vi "Ignore_Channel_evaluate.vi"(7 "Ignore When String":string, 8 "Ignore array":bool[](array[boolean]), 9 "Commands in":string[](array[string]), 10 "Data":string[][](array[string]), 11 "Template Names":string[](array[string])) -> (0 "Ignore array out":bool[](array[boolean]), 1 "Commands Out":string[](array[string]), 3 "Ignore Column":bool)   [LabVIEW 2010]
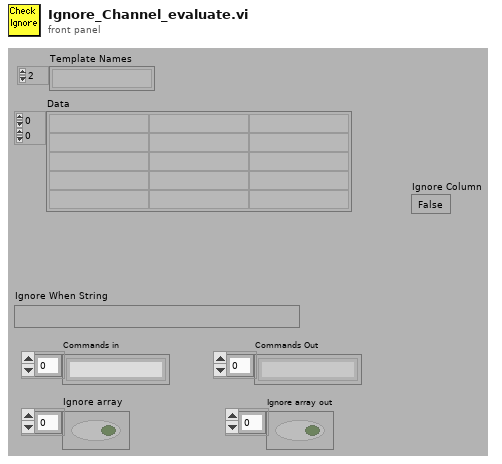
[diagram p1: front panel]
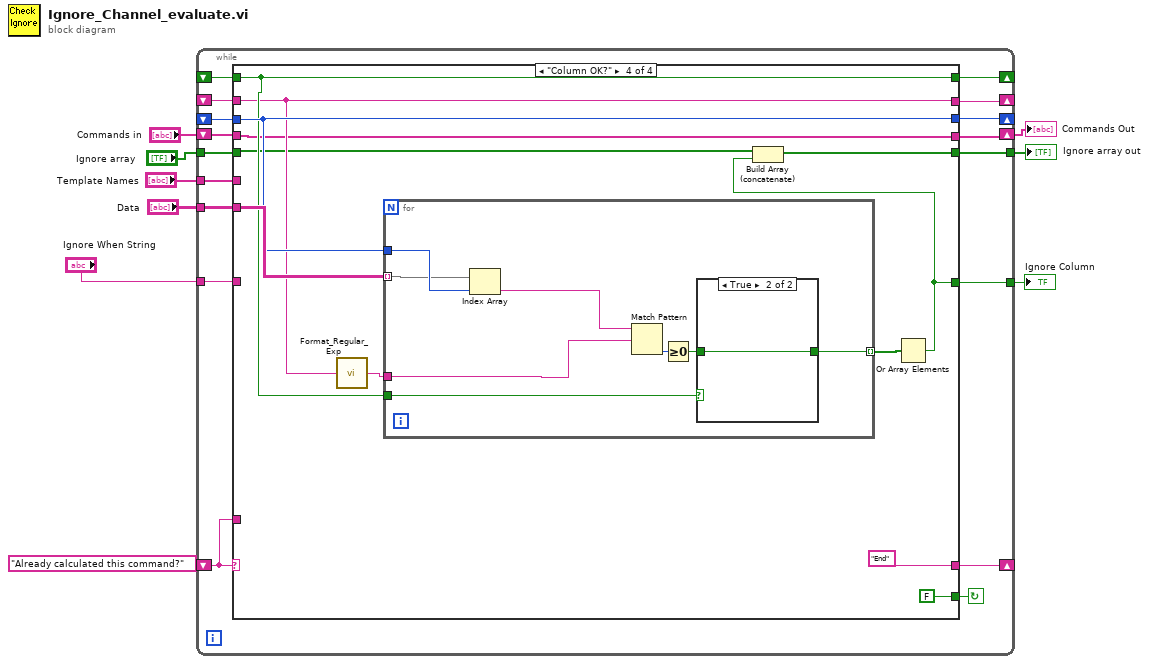
[diagram p0: block diagram]
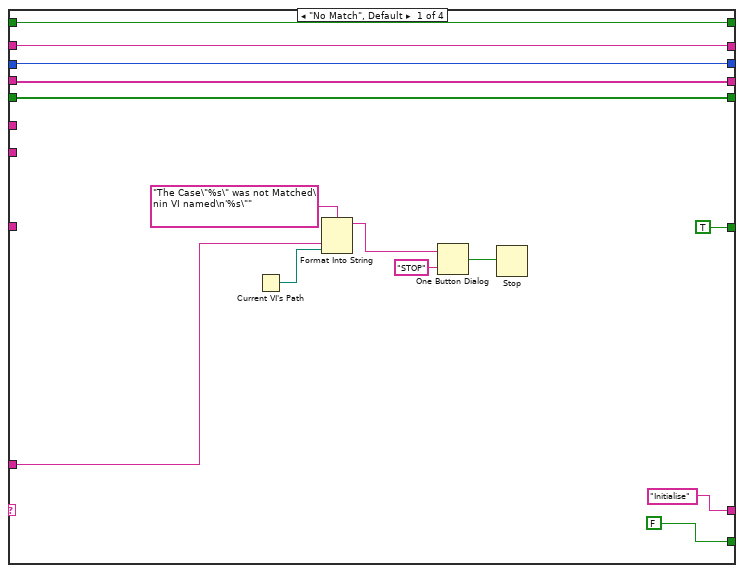
[diagram p2: hidden frame]
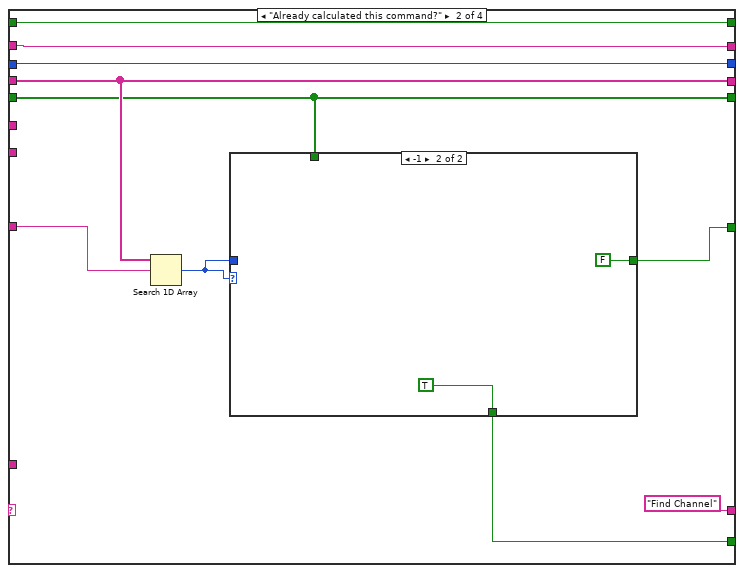
[diagram p3: hidden frame]
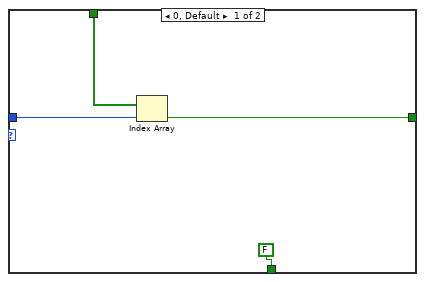
[diagram p4: hidden frame]
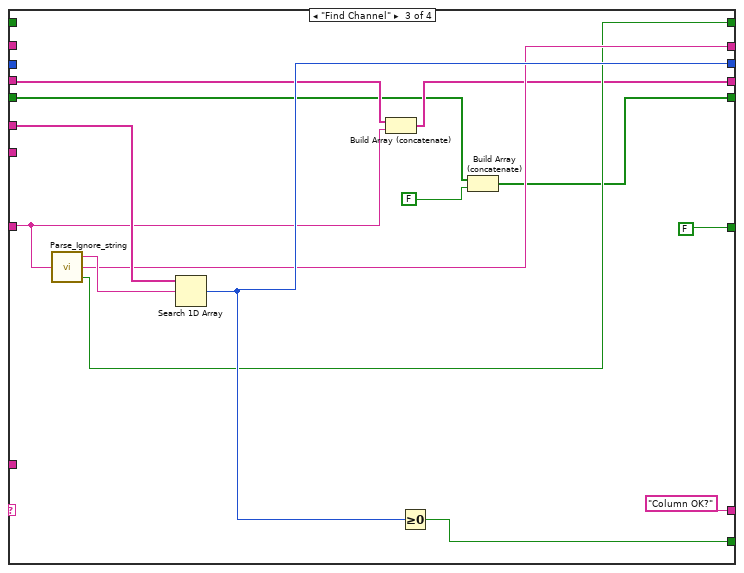
[diagram p5: hidden frame]
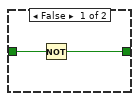
[diagram p6: hidden frame]
diagram:
  n1 = while {
    tunnel: [w19] -> w6
    tunnel: "Data" -> [w21]
    shift-left: _ -> [w20]
    shift-right: [w22] -> _
    tunnel: "Template Names" -> [w23]
    shift-left: "Already calculated this command?" -> [w24]
    shift-right: [w25] -> _
    tunnel: "Ignore When String" -> [w18]
    tunnel: "Ignore array" -> [w17]
    tunnel: [w16] -> w3
    shift-right: [w15] -> _
    shift-left: _ -> [w14]
    shift-right: [w13] -> _
    shift-left: _ -> [w12]
    shift-right: [w10] -> w1
    shift-left: "Commands in" -> [w11]
    stop <- w26 continue-if-true
    n2 = case shown="\"Column OK?\"" w24 {
      tunnel: [FALSE w43 w67 FALSE] -> w26
      tunnel: ["Initialise" "Find Channel" "Column OK?" "End"] -> w25
      tunnel: w24 -> [w35 _ _ _]
      tunnel: w23 -> [_ _ w69 _]
      tunnel: [w32 w49 w68 w78] -> w22
      tunnel: w21 -> [_ _ _ w81]
      tunnel: w20 -> [w32 w49 _ w78]
      tunnel: [TRUE w44 FALSE w71] -> w19
      tunnel: w18 -> [_ w48 w62 _]
      tunnel: w11 -> [w30 w47 w61 w74]
      tunnel: w17 -> [w29 w46 w59 w73]
      tunnel: [w29 w46 w57 w72] -> w16
      tunnel: [w30 w47 w60 w74] -> w10
      tunnel: [w27 w42 w64 w75] -> w15
      tunnel: w14 -> [w27 w42 _ w75]
      tunnel: [w28 w41 w63 w76] -> w13
      tunnel: w12 -> [w28 w41 _ w76]
      frame "No Match", Default {
        n3 = Current VI's Path() -> (path=w34:path)
        n4 = Format Into String(format string="The Case\"%s\" was not Matched\nin VI named\n'%s\"" ("Format String"), w35, w34) -> (resulting string=w38:string)  [unwired: 2 in, 1 out]
        n5 = One Button Dialog(message=w38, button name ("OK")="STOP") -> (true=w36:bool)
        n6 = Stop(stop? (T)=w36) -> ()
      }
      frame "Already calculated this command?" {
        n7 = Search 1D Array(1D array=w47, element=w48) -> (index of element=w45:i32)  [unwired: 1 out]
        n8 = case shown="-1" w45 {
          tunnel: w46 -> [w54 _]
          tunnel: w45 -> [w53 _]
          tunnel: [w52 FALSE ("Boolean")] -> w44
          tunnel: [FALSE TRUE] -> w43
          frame 0, Default {
            n9 = Index Array(array=w54, index=w53) -> (element=w52:bool)
          }
          frame -1 {
          }
        }
      }
      frame "Find Channel" {
        n10 = call "Parse_Ignore_string.vi"("Ignore When String"=w62) -> ("Channel Name"=w65:string, "Search String"=w64:string, "Does Contain"=w63:bool)
        n11 = Search 1D Array(1D array=w69, element=w65) -> (index of element=w68:i32)  [unwired: 1 out]
        n12 = Build Array (concatenate)(w61, w62) -> (w60:string[])
        n13 = Greater Or Equal To 0?(x=w68) -> (x >= 0?=w67:bool)
        n14 = Build Array (concatenate)(w59, FALSE) -> (w57:bool[])
      }
      frame "Column OK?" {
        n15 = call "Format_Regular_Exp.vi"("Regular expression"=w75) -> ("Case Insensitive for html"=w80:string)
        n16 = for {
          tunnel: w81 -> [w86] mode=indexing
          tunnel: w78 -> [w87]
          tunnel: w80 -> [w90]
          tunnel: w76 -> [w89]
          tunnel: [w88] -> w79 mode=indexing
          n17 = Index Array(array=w86, index=w87) -> (element=w85:string)
          n18 = Match Pattern(string=w85, regular expression=w90) -> (offset past match=w84:i32)  [unwired: 4 out]
          n19 = Greater Or Equal To 0?(x=w84) -> (x >= 0?=w83:bool)
          n20 = case shown="True" w89 {
            tunnel: [w91 w93] -> w88
            tunnel: w83 -> [w92 w93]
            frame False {
              n21 = Not(x=w92) -> (.not. x?=w91:bool)
            }
            frame True {
            }
          }
        }
        n22 = Or Array Elements(Boolean array=w79) -> (logical OR=w71:bool)
        n23 = Build Array (concatenate)(w73, w71) -> (w72:bool[])
      }
    }
  }
  "Ignore Column" <- w6
  "Commands Out" <- w1
  "Ignore array out" <- w3
